vi "Read Element of Coefficients.vi"(8 "error in (no error)":errorcluster, 10 "index":i32, 11 "Thruster in":refnum<class "Thruster.lvclass">) -> (0 "error out":errorcluster, 2 "Numeric":dbl, 3 "Thruster out":refnum<class "Thruster.lvclass">)   [LabVIEW 2014, in "Thruster.lvclass"]
uses:
  Thruster.lvclass
  Thruster.lvclass/Thruster.ctl
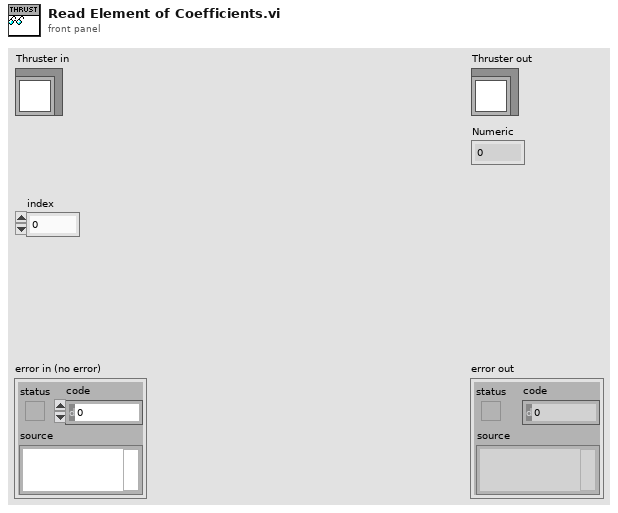
[diagram p1: front panel]
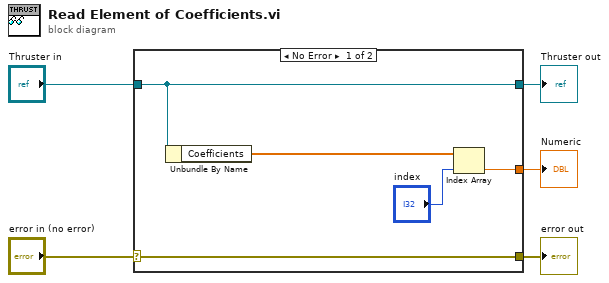
[diagram p0: block diagram]
diagram:
  n1 = case shown="No Error" "error in (no error)" {
    selector: "error in (no error)" -> [w10 w11]
    tunnel: [w10 w11] -> w4
    tunnel: [w9 w12] -> w2
    tunnel: "Thruster in" -> [w9 w12]
    tunnel: [w6 _] -> w1
    frame No Error {
      n2 = Unbundle By Name(w9) -> ("Coefficients"=w8:dbl[])
      n3 = Index Array(array=w8, index="index") -> (element=w6:dbl)
    }
    frame Error {
    }
  }
  "error out" <- w4
  "Thruster out" <- w2
  "Numeric" <- w1
